vi "Select Mask.vi"(6 "error in":errorcluster, 7 "Prompt":string="Select Left Mask", 8 "Read \nImage":T3(plugin-control)=refnum) -> (0 "error out":errorcluster, 1 "Cancelled":bool, 2 "ROI Descriptor Out":T1 {"Contours"."Type" items=["No Selection", "Point", "Line", "Rectangle", "Oval", "Polygon", "Freehand Region", "Annulus", "Unused2", "Unused3", "Broken Line", "Freehand Line", "Rotated Rectangle"]}, 3 "Masked \nImage":T3(plugin-control), 4 "Annulus":T2={"Center X"=982, "Center Y"=650, "Inner Radius"=309, "Outer Radius"=405, "Start Angle"=90.0, "End Angle"=180.0} {"End Angle" format="%.2f"; "Start Angle" format="%.2f"; "Center X" scale=0.0..1024.0}, 5 "mask":T3(plugin-control))   [LabVIEW 2013, in "Image Processing.lvlib"]
uses:
  Image Processing.lvlib
  <vilib>/vision/NI_Vision_Development_Module.lvlib
panel:
  in  "Annulus Angles":cluster{"Start Angle":dbl, "End Angle":dbl}={"Start Angle"=0.0, "End Angle"=90.0}
  in  "Set Window Coordinates":cluster{"X Position":i32, "Y Position":i32}={"X Position"=0, "Y Position"=100}
  out "Window Coordinates":cluster{"X Position":i32, "Y Position":i32}={"X Position"=0, "Y Position"=100}
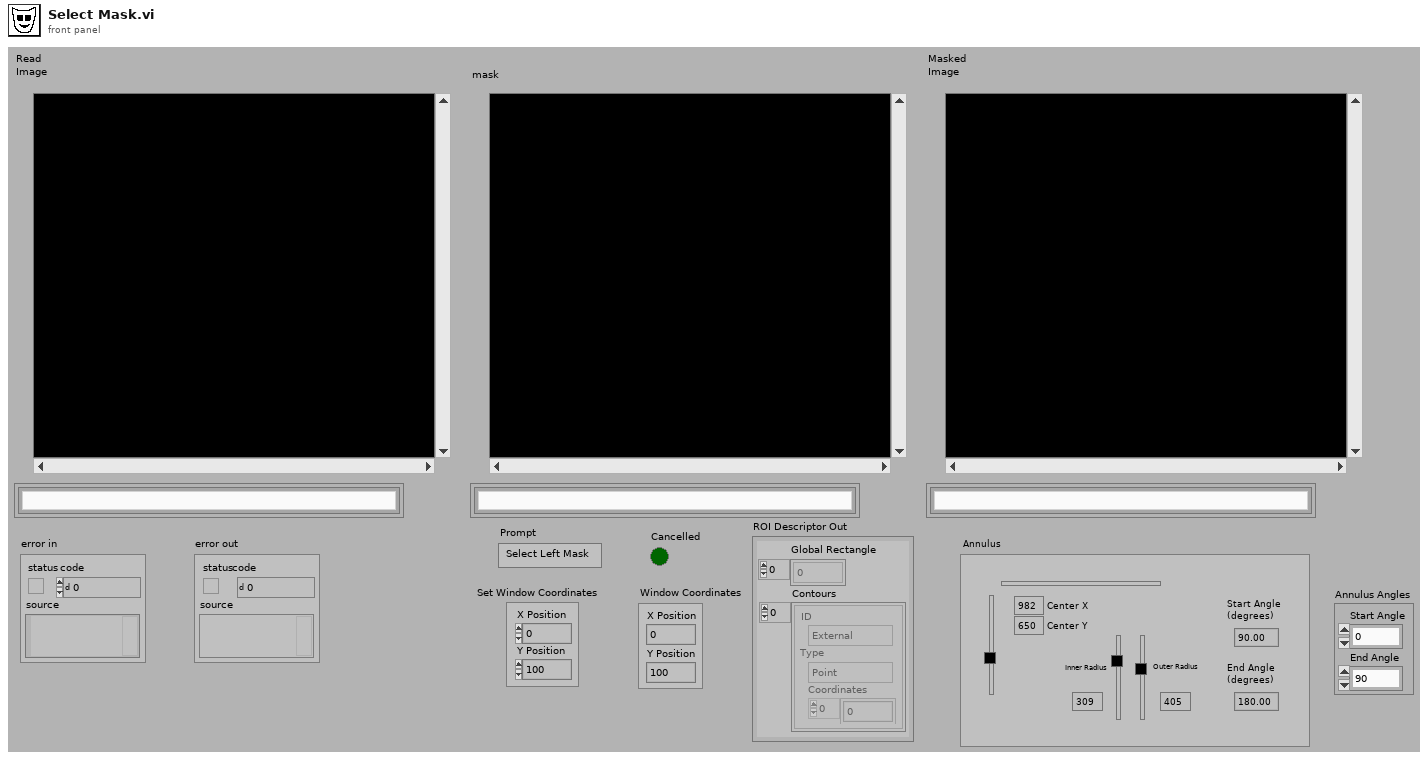
[diagram p1: front panel]
types:
  T1 = typedef "ROI Descriptor" = cluster{"Global Rectangle":i32[], "Contours":cluster{"ID":enum32{"External", "Internal"}, "Type":u32, "Coordinates":i32[]}[]}
  T2 = typedef "IMAQ Circle" = cluster{"Center X":i32, "Center Y":i32, "Inner Radius":i32, "Outer Radius":i32, "Start Angle":dbl, "End Angle":dbl}
  T3 = typedef "IMAQ Image.ctl" = refnum<image>
  T4 = enum32{"Gray", "Binary", "Gradient", "Rainbow", "Temperature"}
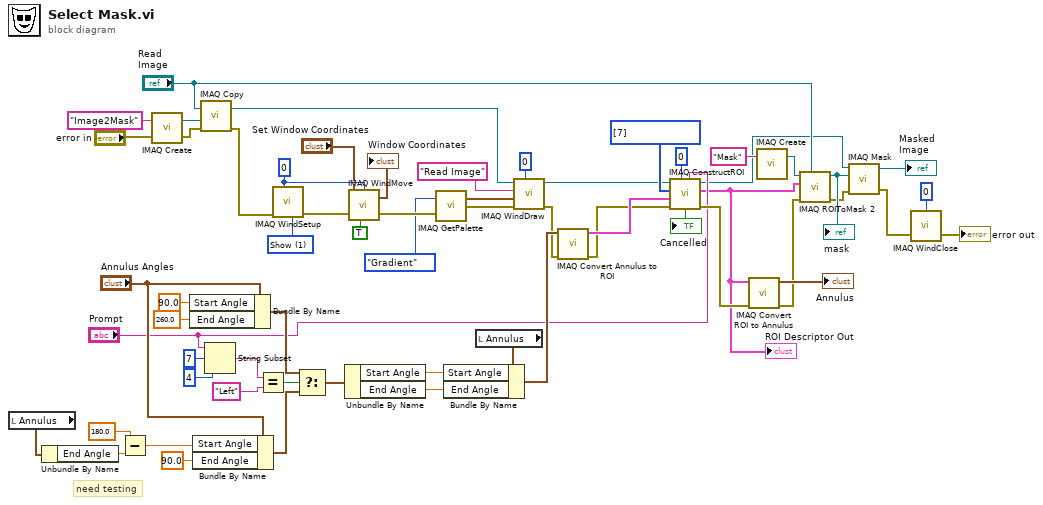
[diagram p0: block diagram]
diagram:
  w18 = u32[] [7] items=["No Selection", "Point", "Line", "Rectangle", "Oval", "Polygon", "Freehand Region", "Annulus", "Zoom", "Pan", "Broken Line", "Freehand Line", "Rotated Rectangle"] ("Tools")
  w52 = 1 items=["Hide", "Show", "No change"] ("Scrollbars (No change)")
  w48 = 0 ("Window Number (0...15)")
  # "need testing"
  n1 = local read "Annulus"() -> (w1:T2)
  n2 = Unbundle By Name(w1) -> ("End Angle"=w3:dbl)
  n3 = Subtract(x=180.0, y=w3) -> (x-y=w2:dbl)
  n4 = call "IMAQ Create"("Image Name"="Image2Mask", "error in (no error)"="error in") -> ("New Image"=w44:T3, "error out"=w40:errorcluster)  [unwired: 3 in]
  n5 = Bundle By Name(cluster="Annulus Angles", "Start Angle"=90.0, "End Angle"=260.0) -> (w28:cluster{"Start Angle":dbl, "End Angle":dbl})
  n6 = Bundle By Name(cluster="Annulus Angles", "Start Angle"=w2, "End Angle"=90.0) -> (w25:cluster{"Start Angle":dbl, "End Angle":dbl})
  n7 = call "IMAQ Copy"("error in (no error)"=w40, "Image Dst"=w44, "Image Src"="Read \nImage") -> ("error out"=w38:errorcluster, "Image Dst Out"=w42:T3)  [unwired: 3 in]
  n8 = String Subset(string="Prompt", offset (0)=7, length (rest)=4 ("length (rest)")) -> (substring=w32:string)
  n9 = Equal?(x=w32, y="Left") -> (x = y?=w31:bool)
  n10 = call "IMAQ WindSetup"("Scrollbars (No change)"=w52, "Window Number (0...15)"=w48, "error in (no error)"=w38) -> ("error out"=w50:errorcluster)  [unwired: 8 in]
  n11 = Select(t=w28, s=w31, f=w25) -> (s? t:f=w24:cluster{"Start Angle":dbl, "End Angle":dbl})
  n12 = Unbundle By Name(w24) -> ("Start Angle"=w23:dbl, "End Angle"=w22:dbl)
  n13 = call "IMAQ WindMove"("Window Number (0...15)"=w48, "Coordinates (screen)"="Set Window Coordinates", "Get/Set Status? (Set)"=TRUE, "error in (no error)"=w50) -> ("Coordinates (screen)"=→"Window Coordinates":cluster{"X Position":i32, "Y Position":i32}, "error out"=w47:errorcluster)  [unwired: 1 in]
  n14 = call "IMAQ GetPalette"("Palette Number (gray)"=T4."Gradient", "error in (no error)"=w47) -> ("Color Palette"=w54:cluster{"Red":u8, "Green":u8, "Blue":u8}[], "error out"=w53:errorcluster)  [unwired: 3 in]
  n15 = local read "Annulus"() -> (w37:T2)
  n16 = Bundle By Name(cluster=w37, "Start Angle"=w23, "End Angle"=w22) -> (w36:T2)
  n17 = call "IMAQ WindDraw"("Window Number (0...15)"=0, "error in (no error)"=w53, "Color Palette"=w54, "Title"="Read Image", "Image"=w42) -> ("error out"=w21:errorcluster, "Image Out (duplicate)"=w15:T3)  [unwired: 1 in, 4 out]
  n18 = call "IMAQ Convert Annulus to ROI"("error in (no error)"=w21, "Annulus"=w36) -> ("error out"=w16:errorcluster, "ROI Descriptor"=w17:T1)  [unwired: 7 in]
  n19 = call "IMAQ ConstructROI"("Prompt"="Prompt", "Window Number (-1...15)"=0 ("Window Number (0...15)"), "error in (no error)"=w16, "ROI Descriptor In (None)"=w17, "Tools"=w18, "Image"=w15) -> ("error out"=w20:errorcluster, "Cancel"=→"Cancelled":bool, "ROI Descriptor Out"=w10:T1, "Image Out (duplicate)"=w13:T3)  [unwired: 2 in]
  "ROI Descriptor Out" <- w10
  n20 = call "IMAQ Convert ROI to Annulus"("error in (no error)"=w20, "ROI Descriptor"=w10) -> ("error out"=w9:errorcluster, "Annulus"=→"Annulus":T2)  [unwired: 7 in]
  n21 = call "IMAQ Create"("Image Name"="Mask") -> ("New Image"=w57:T3)  [unwired: 3 in, 2 out]
  n22 = call "IMAQ ROIToMask 2"("Image Model"="Read \nImage", "error in (no error)"=w9, "ROI Descriptor"=w10, "Image"=w57) -> ("error out"=w56:errorcluster, "Image Out"=w59:T3)  [unwired: 5 in, 1 out]
  "mask" <- w59
  n23 = call "IMAQ Mask"("error in (no error)"=w56, "Image Mask"=w59, "Image Src"=w13) -> ("error out"=w7:errorcluster, "Image Dst Out"=→"Masked \nImage":T3)  [unwired: 1 in, 1 out]
  n24 = call "IMAQ WindClose"("Window Number (0...15)"=0, "error in (no error)"=w7) -> ("error out"=→"error out":errorcluster)  [unwired: 4 in]
